vi "List Classes.vi"(8 "error in (no error)":errorcluster, 11 "Rename in":refnum<class "ProjectItem.lvclass">) -> (0 "error out":errorcluster, 3 "Rename out":refnum<class "ProjectItem.lvclass">)   [LabVIEW 2019, in "ProjectItem.lvclass"]
uses:
  ProjectItem.lvclass
  ProjectItem.lvclass/ProjectItem.ctl
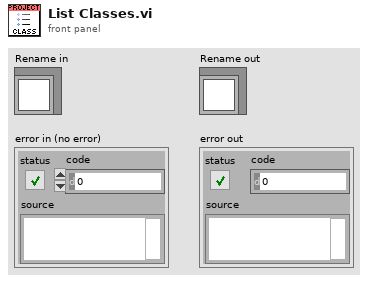
[diagram p1: front panel]
types:
  T1 = cluster{"Class":refnum<vi>, "DynamicVIs":refnum<vi>[], "StaticVIs":refnum<vi>[], "Controls":refnum<vi>[], "Name":string, "Icon":refnum<class "Icon.lvclass">, "Wire Foreground Color":u32}[]
  T2 = cluster{"Class":refnum<vi>, "DynamicVIs":refnum<vi>[], "StaticVIs":refnum<vi>[], "Controls":refnum<vi>[], "Name":string, "Icon":refnum<class "Icon.lvclass">, "Wire Foreground Color":u32}
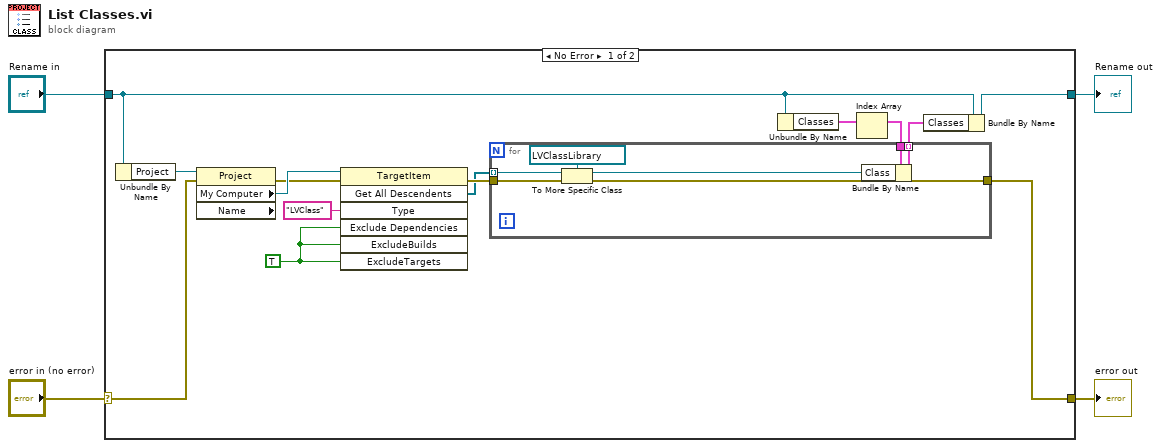
[diagram p0: block diagram]
diagram:
  n1 = case shown="No Error" "error in (no error)" {
    selector: "error in (no error)" -> [w12 w27]
    tunnel: [w18 w26] -> w4
    tunnel: "Rename in" -> [w5 w26]
    tunnel: [w6 w27] -> w2
    frame No Error {
      w15 = TRUE ("ExcludeDependencies")
      n2 = Unbundle By Name(w5) -> ("Project"=w17:refnum<vi>)
      n3 = property class="Project" props=["My Computer", "Name"](reference=w17, error in=w12) -> (error out=w13:errorcluster, "My Computer"=w16:refnum<vi>)  [unwired: 2 out]
      n4 = invoke class="TargetItem" method="Get All Descendents"(reference=w16, error in=w13, "Type"="LVClass", "Exclude Dependencies"=w15, "ExcludeBuilds"=w15, "ExcludeTargets"=w15) -> (error out=w8:errorcluster, "All Descendents"=w7:refnum<vi>[])  [unwired: 1 in, 5 out]
      n5 = Unbundle By Name(w5) -> ("Classes"=w11:T1)
      n6 = Index Array(array=w11) -> (element=w9:T2)  [unwired: 1 in]
      n7 = for {
        tunnel: w9 -> [w25]
        tunnel: [w24] -> w10 mode=indexing
        tunnel: w7 -> [w22] mode=indexing
        tunnel: w8 -> [w21]
        tunnel: [w19] -> w6
        n8 = To More Specific Class(target class=refnum<vi> refnum ("reference"), reference=w22, error in=w21) -> (specific class reference=w20:refnum<vi>, error out=w19:errorcluster)
        n9 = Bundle By Name(cluster=w25, "Class"=w20) -> (w24:T2)
      }
      n10 = Bundle By Name(cluster=w5, "Classes"=w10) -> (w18:refnum<class "ProjectItem.lvclass">)
    }
    frame Error {
    }
  }
  "Rename out" <- w4
  "error out" <- w2
